vi "Embedded Project.vi"() -> ()   [LabVIEW 2015]
uses:
  <vilib>/Instr/_visa.llb/Select Event Type.ctl
  <vilib>/Instr/_visa.llb/VISA Configure Serial Port (Instr).vi
panel:
  in  "Tab Control":enum32{"Main", "Misc"}(tab)
  out "Structure\nWarning":bool
  out "Tsunami \nWarning":bool
  out "Earthquake\nWarning":bool
  out "Bridge Stress":i32[][](graph)
  out "Node 3":bool
  out "Node 2":bool
  out "Node 1":bool
  out "Z Axis":i16[][](graph)
  out "Y Axis":i16[][](graph)
  out "X Axis":i16[][](graph)
  out "Node 1 level":u8(slide) scale=0.0..3.0
  out "Node 2 level":u8(slide) scale=0.0..3.0
  out "Node 3 level":u8(slide) scale=0.0..3.0
  out "Serial Monitor":string
  in  "COM Port":refnum<visa-resource-name>="COM1"
  out "Array":cluster{"Node Address":u16, "Value":u16}[](array[cluster])
  in  "stop":bool
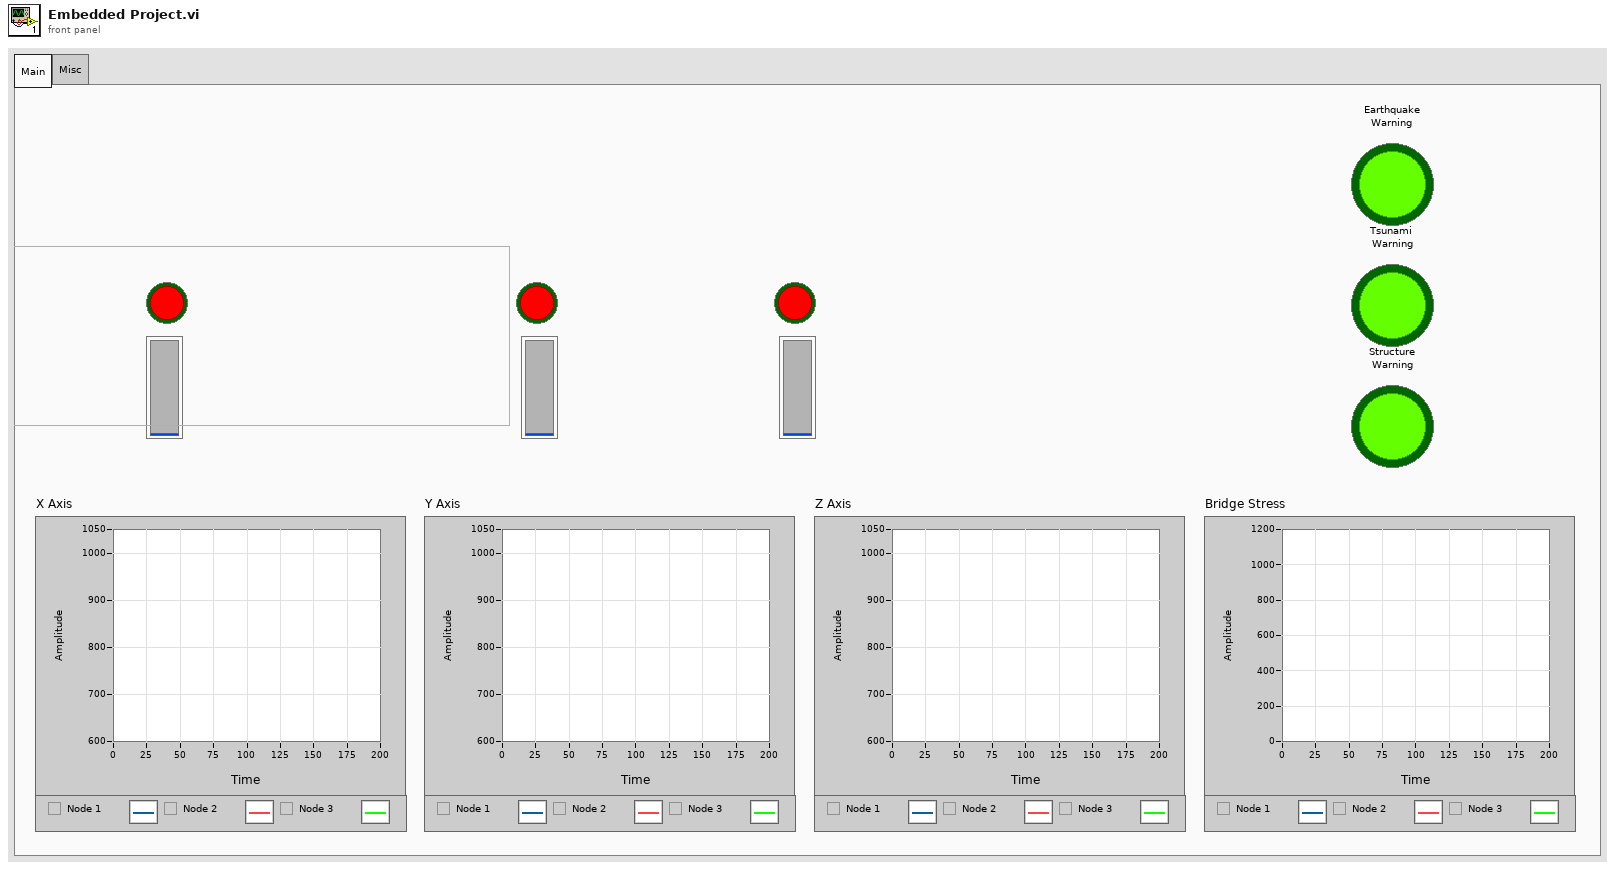
[diagram p1: front panel]
types:
  T1 = cluster{"Node Address":u16, "X Axis":i16, "Y Axis":i16, "Z Axis":i16, "Load Cell":dbl, "Water Level":u8}
  T2 = typedef "Select Event Type.ctl" = u32
  T3 = cluster{"baud rate (9600)":u32, "data bits (8)":u16, "parity (0:none)":enum16{"None", "Odd", "Even", "Mark", "Space"}, "stop bits (10: 1 bit)":u16, "flow control (0:none)":u16}
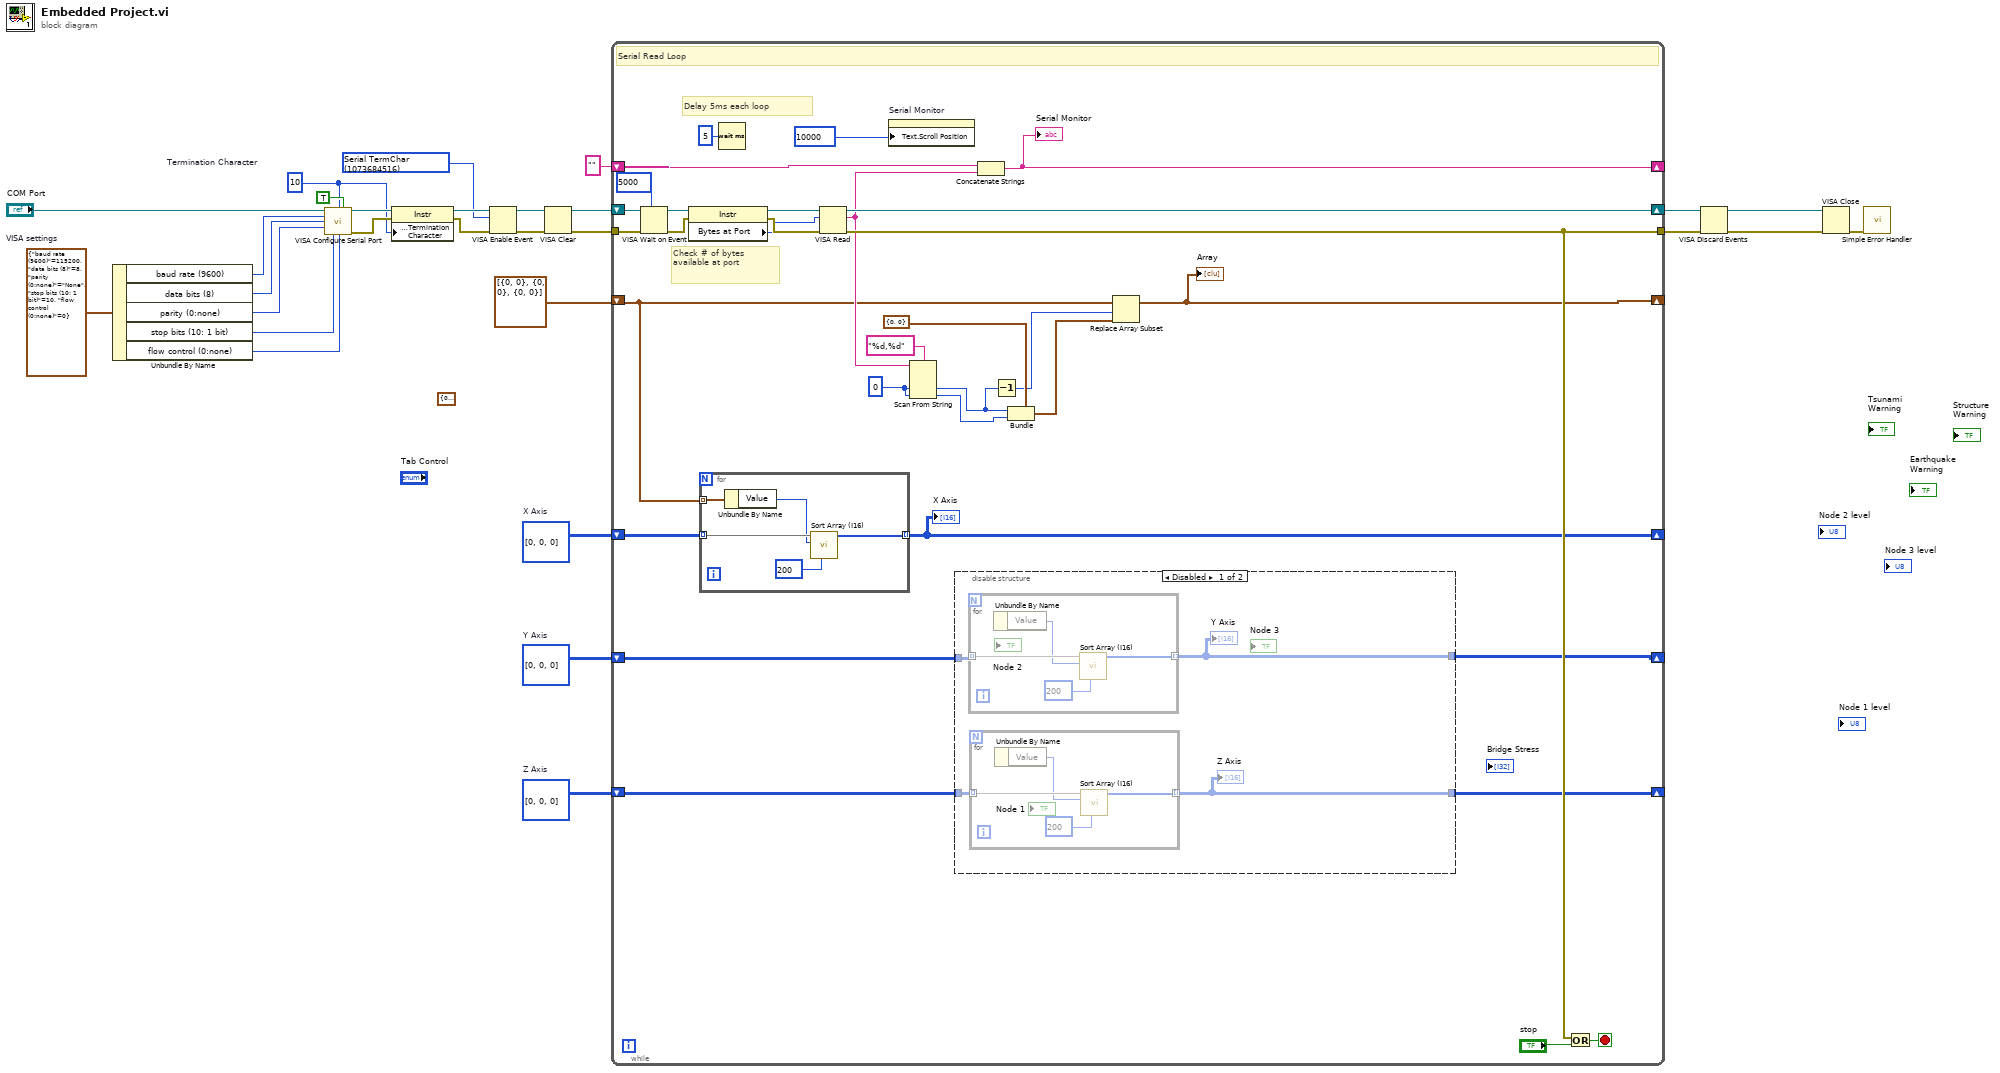
[diagram p0: block diagram]
diagram:
  w1 = u16[][] [[0], [0], [0]]  # Z Axis
  w2 = u16[][] [[0], [0], [0]]  # Y Axis
  (unwired) T1 {"Node Address"=0, "X Axis"=0, "Y Axis"=0, "Z Axis"=0, "Load Cell"=0.0, "Water Level"=0} ("Node 1")
  w3 = u16[][] [[0], [0], [0]]  # X Axis
  w14 = T2 1073684516 items=["Service Request"=1073684491, "Trigger"=3221168138, "Clear"=1073684493, "VXI Signal"=1073684512, "VXI/VME Interrupt"=3221168161, "VXI/VME Sysfail"=1073684509, "VXI/VME Sysreset"=1073684510, "GPIB CIC"=1073684498, "GPIB Talk"=1073684499, "GPIB Listen"=1073684500, "PXI Interrupt"=1073684514, "Serial Break"=1073684515, "Serial TermChar"=1073684516, "Serial CTS"=1073684521, "Serial DSR"=1073684522, "Serial DCD"=1073684524, "Serial RI"=1073684526, "Serial Character"=1073684533, "USB Interrupt"=1073684535, "All Enabled"=1073709055] ("Event Type")
  w24 = T3 {"baud rate (9600)"=115200, "data bits (8)"=8, "parity (0:none)"=enum."None", "stop bits (10: 1 bit)"=10, "flow control (0:none)"=0}  # VISA settings
  w17 = u8 10  # Termination Character
  n1 = Unbundle By Name(w24) -> ("baud rate (9600)"=w23:u32, "data bits (8)"=w22:u16, "parity (0:none)"=w21:enum16{"None", "Odd", "Even", "Mark", "Space"}, "stop bits (10: 1 bit)"=w20:u16, "flow control (0:none)"=w19:u16)
  n2 = call-poly "VISA Configure Serial Port"("VISA resource name"="COM Port", "termination char\n(0xA = '\\n' = LF)"=w17, "Enable Termination\nChar (T)"=TRUE ("End Read on Termination Character?"), "baud rate (9600)"=w23, "data bits (8)"=w22, "parity (0:none)"=w21, "stop bits (10: 1 bit)"=w20, "flow control (0:none)"=w19) -> ("VISA resource name out"=w27:refnum<visa-resource-name>, "error out"=w18:errorcluster)  [unwired: 2 in, 4 out]
  n3 = property class="Instr"(reference=w27, error in=w18, "Message Based Settings:Termination Character"=w17) -> (reference out=w15:refnum<visa-resource-name>, error out=w16:errorcluster)
  n4 = VISA Enable Event(8:w16, 10:w14, 11:w15) -> (0:w10:errorcluster, 3:w12:refnum<visa-resource-name>)  [unwired: 1 in]
  n5 = VISA Clear(VISA resource name=w12, error in (no error)=w10) -> (VISA resource name out=w11:refnum<visa-resource-name>, error out=w9:errorcluster)
  n6 = while {
    shift-right: [w60] -> w8
    shift-left: w11 -> [w53]
    tunnel: [w57] -> w5
    shift-right: [w54] -> _
    shift-left: "" -> [w55]
    tunnel: w9 -> [w52]
    shift-right: [w38] -> _
    shift-left: cluster{"Node Address":u16, "Value":u16}[] [{"Node Address"=0, "Value"=0}, {"Node Address"=0, "Value"=0}, {"Node Address"=0, "Value"=0}] ("Array") -> [w36]
    shift-right: [w34] -> _
    shift-left: w3 -> [w35]
    shift-right: [w33] -> _
    shift-left: w2 -> [w32]
    shift-right: [w30] -> _
    shift-left: w1 -> [w31]
    stop <- w58 stop-if-true
    w42 = u16 0 ("default value 1")
    # "Check # of bytes \navailable at port"
    # "Delay 5ms each loop"
    # "Serial Read Loop"
    n7 = VISA Wait on Event(7:u32 5000 ("timeout (0)"), 8:w52, 11:w53) -> (0:w50:errorcluster, 3:w51:refnum<visa-resource-name>)  [unwired: 2 in, 2 out]
    n8 = property class="Instr"(reference=w51, error in=w50) -> (reference out=w49:refnum<visa-resource-name>, error out=w48:errorcluster, "Bytes at Port"=w47:u32)
    n9 = for {
      tunnel: w36 -> [w77] mode=indexing
      tunnel: w35 -> [w76] mode=indexing
      tunnel: [w74] -> w34 mode=indexing
      n10 = Unbundle By Name(w77) -> ("Value"=w75:u16)
      n11 = call "Sort Array (I16).vi"("Max Size"=200, "New Element"=w75, "Array In"=w76) -> ("Array Out"=w74:i16[])  [unwired: 8 in]
    }
    "X Axis" <- w34
    n12 = Wait (ms)(milliseconds to wait=u32 5) -> ()  [unwired: 1 out]
    n13 = VISA Read(VISA resource name=w49, byte count=w47, error in (no error)=w48) -> (VISA resource name out=w60:refnum<visa-resource-name>, read buffer=w41:string, error out=w57:errorcluster)  [unwired: 1 out]
    n14 = property on="Serial Monitor" class="Str"("Text.Scroll Position"=u32 10000) -> ()  [unwired: 2 in, 2 out]
    n15 = Scan From String(format string="%d,%d", input string=w41, default 1=w42, default 2=w42) -> (output 1=w40:u16, output 2=w44:u16)  [unwired: 2 in, 3 out]
    n16 = disable-structure shown="Disabled" {
      disable-tunnel: [w61 _] -> w33
      disable-tunnel: w32 -> [w64 _]
      disable-tunnel: w31 -> [w63 _]
      disable-tunnel: [w62 _] -> w30
      frame Disabled {
        n17 = for {
          tunnel: w64 -> [w72] mode=indexing
          tunnel: [w71] -> w61 mode=indexing
          n18 = Unbundle By Name() -> ("Value"=w69:u16)  [unwired: 1 in]
          n19 = call "Sort Array (I16).vi"("Max Size"=200, "New Element"=w69, "Array In"=w72) -> ("Array Out"=w71:i16[])  [unwired: 8 in]
        }
        "Y Axis" <- w61
        n20 = for {
          tunnel: [w68] -> w62 mode=indexing
          tunnel: w63 -> [w66] mode=indexing
          n21 = Unbundle By Name() -> ("Value"=w65:u16)  [unwired: 1 in]
          n22 = call "Sort Array (I16).vi"("Max Size"=200, "New Element"=w65, "Array In"=w66) -> ("Array Out"=w68:i16[])  [unwired: 8 in]
        }
        "Z Axis" <- w62
      }
      frame Enabled {
      }
    }
    n23 = Concatenate Strings(w55, w41) -> (w54:string)
    "Serial Monitor" <- w54
    n24 = Decrement(x=w40) -> (x-1=w39:u16)
    n25 = Bundle(cluster=cluster{"Node Address":u16, "Value":u16} {"Node Address"=0, "Value"=0} ("Node 1"), "Node Address"=w40, "Value"=w44) -> (w37:cluster{"Node Address":u16, "Value":u16})
    n26 = Replace Array Subset(array=w36, new element=w37, index=w39) -> (w38:cluster{"Node Address":u16, "Value":u16}[])
    "Array" <- w38
    n27 = Or(x=w57, y="stop") -> (x .or. y?=w58:bool)
  }
  n28 = VISA Discard Events(8:w5, 11:w8) -> (0:w6:errorcluster, 3:w7:refnum<visa-resource-name>)  [unwired: 2 in]
  n29 = VISA Close(VISA resource name=w7, error in (no error)=w6) -> (error out=w25:errorcluster)
  n30 = call <vilib>:"Simple Error Handler.vi"("error in (no error)"=w25) -> ()  [unwired: 1 in, 8 out]
